vi "Show FP.vi"(8 "error in (no error)":errorcluster) -> (0 "error out":errorcluster)   [LabVIEW 2018, in "Fuel Farm.lvlib"]
doc: "This subVI enqueues the named action in to the communications queue along with the input data."
uses:
  Fuel Farm.lvlib
  Private Controls/Module Data.ctl
  Private Controls/Module Action.ctl
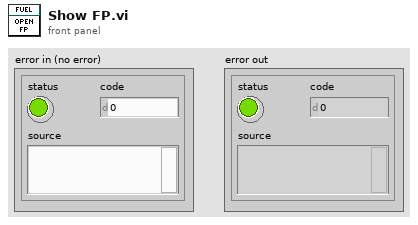
[diagram p1: front panel]
types:
  T1 = typedef "Fuel Farm.lvlib/Module Data.ctl" = cluster{"Data":variant, "Action":T2}
  T2 = typedef "Fuel Farm.lvlib/Module Action.ctl" = enum8{"Init", "Open FP", "Timeout", "Error", "Exit"}
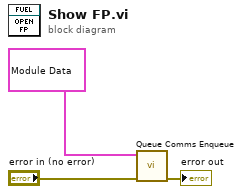
[diagram p0: block diagram]
diagram:
  n1 = call "Queue Comms Enqueue.vi"("error in (no error)"="error in (no error)", "element"=T1 {"Data"=variant, "Action"=enum."Open FP"}) -> ("error out"=→"error out":errorcluster)  [unwired: 9 in]
